vi "RPC Method GreeterService GetFeature.vi"(3 "error in (no error)":errorcluster, 4 "gRPCid in":T1, 5 "DNL_LabVIEW Object in":refnum<class "GreeterServiceImpl.lvclass">) -> (0 "error out":errorcluster, 1 "gRPCid out":T1, 2 "DNL_LabVIEW Object out":refnum<class "GreeterServiceImpl.lvclass">)   [LabVIEW 2019, in "UserCode_impl_server.lvlib" / "GreeterServiceImpl.lvclass"]
uses:
  GreeterServiceImpl.lvclass
  <vilib>/gRPC/LabVIEW gRPC Library/Shared/grpcId.ctl
  Generated_stub_server/RPC Messages/Greeter_res.ctl
  Generated_stub_server/RPC Messages/Greeter_res_res_oneof/Greeter_res_res_oneof.lvclass
  Generated_stub_server/RPC Messages/Greeter_req_req_oneof/Greeter_req_req_oneof.lvclass/Greeter_req_req_oneof.ctl
  Generated_stub_server/RPC Messages/Greeter_res_res_oneof/Greeter_res_res_oneof.lvclass/Greeter_res_res_oneof.ctl
  Generated_stub_server/Generated_stub_server.lvlib
  Generated_stub_server/RPC Messages/Greeter_req_req_oneof/Greeter_req_req_oneof.lvclass
  Generated_stub_server/RPC Service/GreeterServiceStub/GreeterServiceStub.lvclass
  <vilib>/gRPC/LabVIEW gRPC Library/grpc-lvsupport-release.lvlib
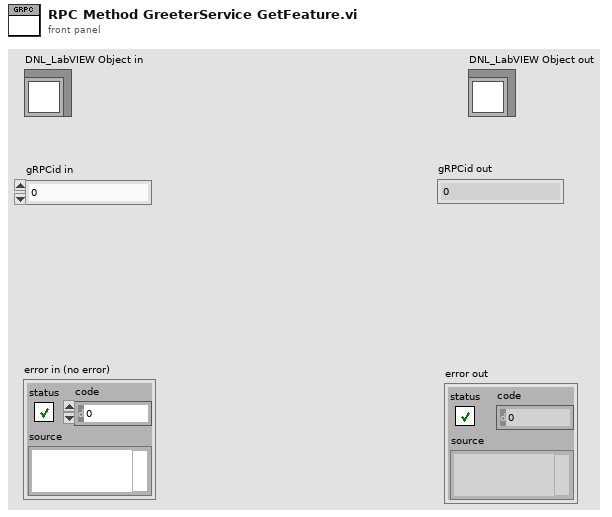
[diagram p1: front panel]
types:
  T1 = typedef "grpc-lvsupport-release.lvlib/grpcId.ctl" = u64
  T2 = typedef "Generated_stub_server.lvlib/Greeter_res.ctl" = cluster{"res_latitude":i32, "Greeter_res_res_oneof":refnum<class "Greeter_res_res_oneof.lvclass">}
  T3 = typedef "Generated_stub_server.lvlib/Greeter_req.ctl" = cluster{"req_latitude":i32, "Greeter_req_req_oneof":refnum<class "Greeter_req_req_oneof.lvclass">}
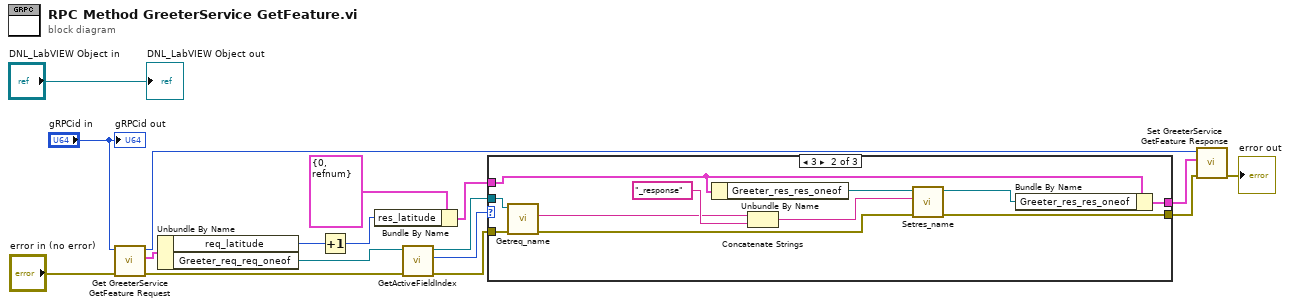
[diagram p0: block diagram]
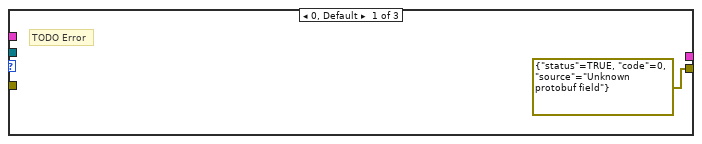
[diagram p2: hidden frame]
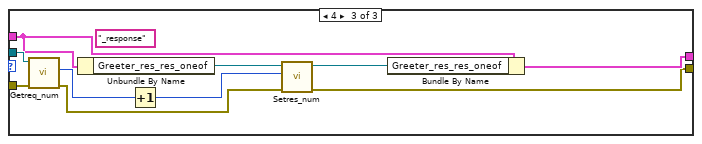
[diagram p3: hidden frame]
diagram:
  n1 = call "Get GreeterService GetFeature Request.vi"("error in (no error)"="error in (no error)", "gRPCid"="gRPCid in") -> ("error out"=w11:errorcluster, "Message Data"=w16:T3, "gRPCid out"=w17:T1)  [unwired: 7 in]
  n2 = Unbundle By Name(w16) -> ("req_latitude"=w14:i32, "Greeter_req_req_oneof"=w12:refnum<class "Greeter_req_req_oneof.lvclass">)
  n3 = Increment(x=w14) -> (x+1=w13:i32)
  n4 = Bundle By Name(cluster=T2 {"res_latitude"=0, "Greeter_res_res_oneof"=refnum} ("Message Data"), "res_latitude"=w13) -> (w7:T2)
  n5 = call "GetActiveFieldIndex.vi"("error in (no error)"=w11, "OneOfTemplate in"=w12) -> ("error out"=w8:errorcluster, "Active Field Index"=w10:i32, "OneOfTemplate out"=w9:refnum<class "Greeter_req_req_oneof.lvclass">)  [unwired: 7 in]
  n6 = case shown="3" w10 {
    tunnel: w9 -> [_ w29 w39]
    tunnel: w8 -> [_ w28 w38]
    tunnel: w7 -> [_ w26 w36]
    tunnel: [_ w21 w34] -> w6
    tunnel: [errorcluster {"status"=TRUE, "code"=0, "source"="Unknown protobuf field"} ("error out") w19 w30] -> w5
    frame 0, Default {
      # "TODO Error"
    }
    frame 3 {
      n7 = call "Getreq_name.vi"("error in (no error)"=w28, "OneOfTemplate in"=w29) -> ("error out"=w20:errorcluster, "Get_Val"=w23:string)  [unwired: 7 in, 1 out]
      n8 = Unbundle By Name(w26) -> ("Greeter_res_res_oneof"=w25:refnum<class "Greeter_res_res_oneof.lvclass">)
      n9 = Concatenate Strings(w23, "_response") -> (w22:string)
      n10 = call "Setres_name.vi"("error in (no error)"=w20, "Set_Val"=w22, "OneOfTemplate in"=w25) -> ("error out"=w19:errorcluster, "OneOfTemplate out"=w27:refnum<class "Greeter_res_res_oneof.lvclass">)  [unwired: 7 in]
      n11 = Bundle By Name(cluster=w26, "Greeter_res_res_oneof"=w27) -> (w21:T2)
    }
    frame 4 {
      (unwired) "_response"
      n12 = call "Getreq_num.vi"("error in (no error)"=w38, "OneOfTemplate in"=w39) -> ("error out"=w31:errorcluster, "Get_Val"=w33:i32)  [unwired: 7 in, 1 out]
      n13 = Unbundle By Name(w36) -> ("Greeter_res_res_oneof"=w35:refnum<class "Greeter_res_res_oneof.lvclass">)
      n14 = Increment(x=w33) -> (x+1=w32:i32)
      n15 = call "Setres_num.vi"("error in (no error)"=w31, "Set_Val"=w32, "OneOfTemplate in"=w35) -> ("error out"=w30:errorcluster, "OneOfTemplate out"=w37:refnum<class "Greeter_res_res_oneof.lvclass">)  [unwired: 7 in]
      n16 = Bundle By Name(cluster=w36, "Greeter_res_res_oneof"=w37) -> (w34:T2)
    }
  }
  n17 = call "Set GreeterService GetFeature Response.vi"("error in (no error)"=w5, "Message Data"=w6, "gRPCid in"=w17) -> ("error out"=→"error out":errorcluster)  [unwired: 8 in]
  "DNL_LabVIEW Object out" <- "DNL_LabVIEW Object in"
  "gRPCid out" <- "gRPCid in"
